vi "Read Data.vi"(8 "error in (no error)":errorcluster, 11 "ITC 503 in":refnum<class "ITC 503.lvclass">) -> (0 "error out":errorcluster, 2 "Data":waveform(dbl)[](array[waveform]), 3 "ITC 503 out":refnum<class "ITC 503.lvclass">)   [LabVIEW 2015, in "ITC 503.lvclass"]
uses:
  ITC 503.lvclass
  Controls/ITC503 FP Data.ctl
  OO Devices/Device/Read Controls Snapshot.vi
  Instrument/Read VISA Resource.vi
  OO Devices/Device/Read Control Panel Loaded.vi
  Instrument/Write VISA Resource.vi
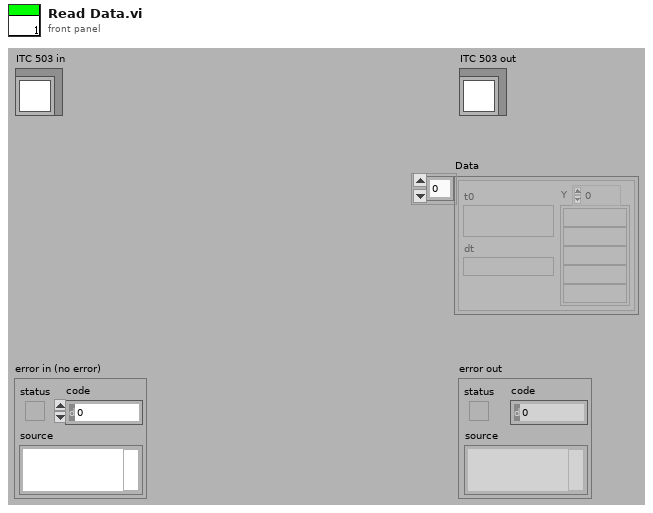
[diagram p1: front panel]
types:
  T1 = typedef "ITC503 FP Data.ctl" = cluster{"Channels to measure":i32[]}
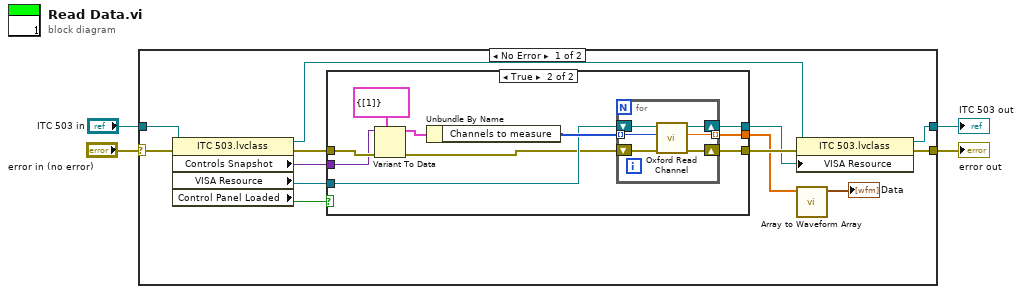
[diagram p0: block diagram]
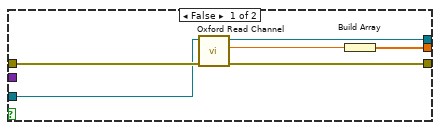
[diagram p2: hidden frame]
diagram:
  n1 = case shown="No Error" "error in (no error)" {
    selector: "error in (no error)" -> [w12 w41]
    tunnel: [w13 w41] -> w3
    tunnel: [w16 w40] -> w1
    tunnel: "ITC 503 in" -> [w17 w40]
    frame No Error {
      n2 = property class="ITC 503.lvclass"(reference=w17, error in=w12) -> (reference out=w6:refnum<class "ITC 503.lvclass">, error out=w11:errorcluster, "Controls Snapshot"=w10:variant, "VISA Resource"=w7:refnum<visa-resource-name>, "Control Panel Loaded"=w5:bool)
      n3 = case shown="True" w5 {
        tunnel: [w22 w33] -> w15
        tunnel: w11 -> [w23 w32]
        tunnel: w10 -> [_ w31]
        tunnel: [w19 w28] -> w9
        tunnel: [w18 w26] -> w8
        tunnel: w7 -> [w21 w25]
        frame False {
          n4 = call "Oxford Read Channel.vi"("error in (no error)"=w23, "VISA resource name"=w21) -> ("error out"=w22:errorcluster, "Data"=w20:dbl, "VISA resource name out"=w18:refnum<visa-resource-name>)  [unwired: 6 in, 1 out]
          n5 = Build Array(w20) -> (w19:dbl[])
        }
        frame True {
          n6 = Variant To Data(error in=w32, type=T1 {"Channels to measure"=[1]} ("Data"), Variant=w31) -> (data=w29:T1, error out=w24:errorcluster)
          n7 = Unbundle By Name(w29) -> ("Channels to measure"=w27:i32[])
          n8 = for {
            tunnel: [w35] -> w28 mode=indexing
            shift-right: [w36] -> w33
            shift-left: w24 -> [w38]
            tunnel: w27 -> [w34] mode=indexing
            shift-right: [w37] -> w26
            shift-left: w25 -> [w39]
            n9 = call "Oxford Read Channel.vi"("error in (no error)"=w38, "Channel #"=w34, "VISA resource name"=w39) -> ("error out"=w36:errorcluster, "Data"=w35:dbl, "VISA resource name out"=w37:refnum<visa-resource-name>)  [unwired: 5 in, 1 out]
          }
        }
      }
      n10 = property class="ITC 503.lvclass"(reference=w6, error in=w15, "VISA Resource"=w8) -> (reference out=w16:refnum<class "ITC 503.lvclass">, error out=w13:errorcluster)
      n11 = call "Array to Waveform Array.vi"("Array"=w9) -> ("Waveform"=→"Data":waveform(dbl)[])  [unwired: 10 in]
    }
    frame Error {
    }
  }
  "error out" <- w3
  "ITC 503 out" <- w1
